vi "Configure.vi"(8 "error in (no error)":errorcluster, 11 "Laser_Oxxius in":refnum<class "Laser_Oxxius.lvclass">) -> (0 "error out":errorcluster, 3 "Laser_Oxxius out":refnum<class "Laser_Oxxius.lvclass">)   [LabVIEW 2020, in "Laser_Oxxius.lvlib" / "Laser_Oxxius.lvclass"]
uses:
  Laser_Oxxius.lvclass
  Laser_Oxxius.lvclass/Laser_Oxxius.ctl
  Hardware Abstraction Layer/Component/Laser/Laser/Laser.lvclass
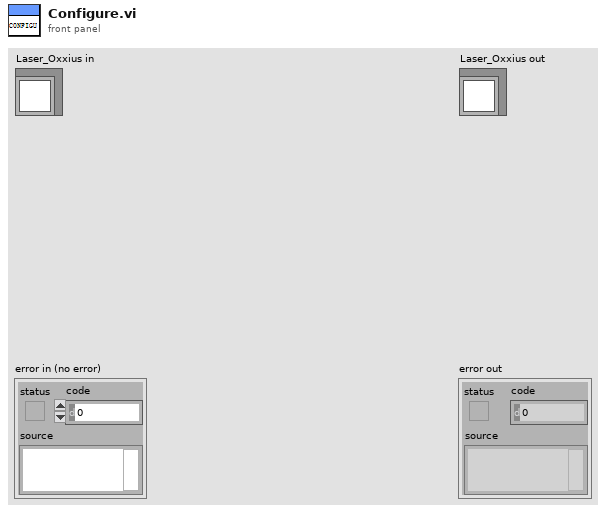
[diagram p1: front panel]
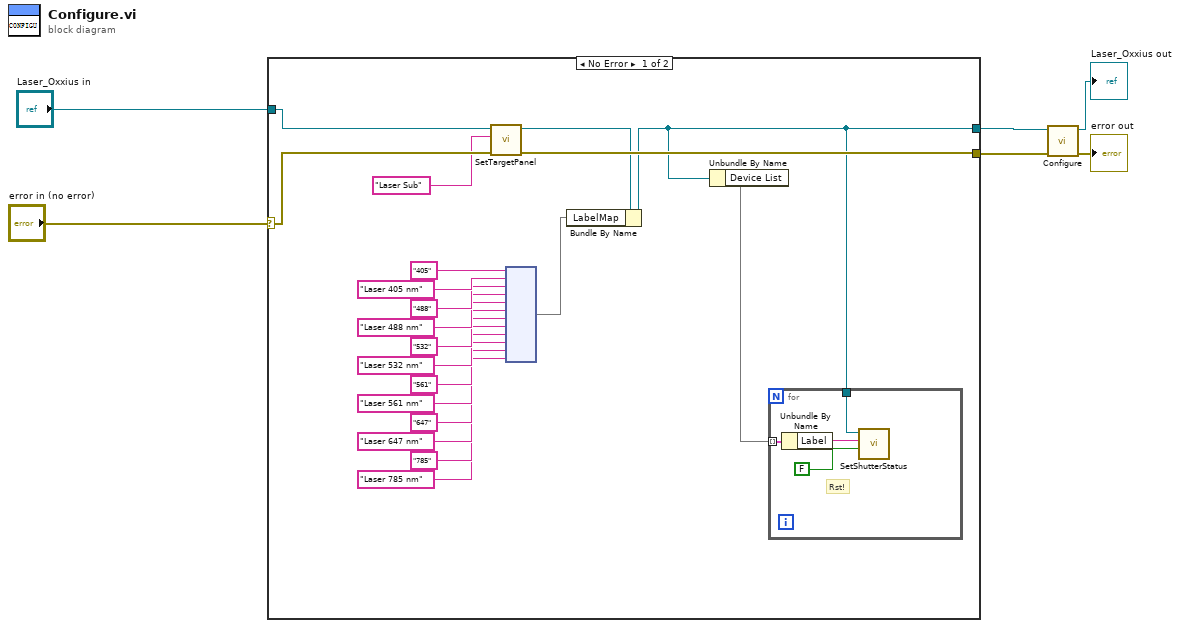
[diagram p0: block diagram]
diagram:
  n1 = case shown="No Error" "error in (no error)" {
    selector: "error in (no error)" -> [w25 w32]
    tunnel: [w24 w32] -> w1
    tunnel: [w8 w31] -> w2
    tunnel: "Laser_Oxxius in" -> [w26 w31]
    frame No Error {
      n2 = call-dynamic "SetTargetPanel.vi"("error in (no error)"=w25, "TargetPanel"="Laser Sub" ("Sub Panel"), "GRMActor in"=w26) -> ("error out"=w24:errorcluster, "GRMActor out"=w22:refnum<class "Laser_Oxxius.lvclass">)  [unwired: 7 in]
      n3 = node("405" ("key"), "Laser 405 nm" ("key"), "488" ("key"), "Laser 488 nm" ("value"), "532" ("key"), "Laser 532 nm" ("value"), "561" ("key"), "Laser 561 nm" ("value"), "647" ("key"), "Laser 647 nm" ("value"), "785" ("key"), "Laser 785 nm" ("value")) -> (w7:map{string, string})
      n4 = Bundle By Name(cluster=w22, "LabelMap"=w7) -> (w8:refnum<class "Laser_Oxxius.lvclass">)
      n5 = Unbundle By Name(w8) -> ("Device List"=w21:map{string, refnum<k24>})
      n6 = for {
        tunnel: w21 -> [w30] mode=indexing
        tunnel: w8 -> [w28]
        # "Rst!"
        n7 = Unbundle By Name(w30) -> ("Label"=w29:string)
        n8 = call-dynamic "SetShutterStatus.vi"("Value"=FALSE, "Label"=w29, "Laser_Oxxius in"=w28) -> ()  [unwired: 7 in, 2 out]
      }
    }
    frame Error {
    }
  }
  n9 = call-parent "Configure.vi"("error in (no error)"=w1, "Device in"=w2) -> ("error out"=→"error out":errorcluster, "Device out"=→"Laser_Oxxius out":refnum<class "Laser_Oxxius.lvclass">)  [unwired: 8 in]
